vi "Set X Channel for XY.vi"(8 "error in (no error)":errorcluster, 10 "Channel for X":u16(ring) items=["A1"=0, "A2"=1, "A3"=2, "A4"=3, "A5"=4, "A6"=5, "A7"=6, "A8"=7, "A9"=8, "A10"=9, "K1"=200, "K2"=201, "K3"=202, "K4"=203, "FA1"=204, "FA2"=205, "FA3"=206, "FA4"=207], 11 "VISA resource name":refnum<visa-resource-name>) -> (0 "error out":errorcluster, 3 "VISA resource name out":refnum<visa-resource-name>)   [LabVIEW 2017, in "Sefram DAS220.lvlib"]
doc: "Set the X channel for XY graph."
uses:
  <instrlib>/Sefram DAS220/Sefram DAS220.lvlib
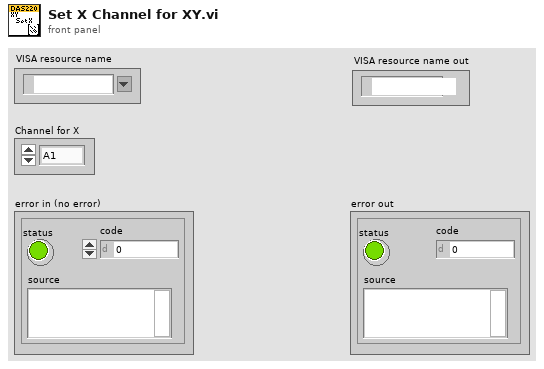
[diagram p1: front panel]
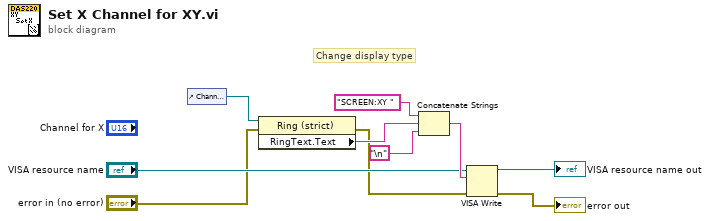
[diagram p0: block diagram]
diagram:
  # "Change display type"
  n1 = control-ref of="Channel for X"() -> (w1:refnum<vi>)
  n2 = property class="Ring (strict)"(reference=w1, error in="error in (no error)") -> (error out=w2:errorcluster, "RingText.Text"=w4:string)  [unwired: 1 out]
  n3 = Concatenate Strings("SCREEN:XY " ("string"), w4, "\n") -> (w10:string)
  n4 = VISA Write(VISA resource name="VISA resource name", write buffer=w10, error in (no error)=w2) -> (VISA resource name out=→"VISA resource name out":refnum<visa-resource-name>, error out=→"error out":errorcluster)  [unwired: 1 out]
